vi "Dashboard Main.vi"() -> ()   [LabVIEW 2012]
uses:
  <vilib>/event_ctls.llb/eventvkey.ctl
  <vilib>/Utility/config.llb/Read Key (String).vi
  <vilib>/Utility/config.llb/Read Key (I32).vi
  <vilib>/Utility/config.llb/Write Key (String).vi
  <vilib>/Utility/config.llb/Write Key (I32).vi
  <vilib>/Utility/config.llb/NI_LVConfig.lvlib
panel:
  out "Mode":T1(ring)=enum."Auto Disabled"
  in  "Viewer":enum32{"Camera Image", "Variables"}(tab)
  out "Mbps":dbl format="%#.1g"
  in  "Enable":bool
  in  "DB Camera Config":bool
  out "Mbps":bool
  out "fps":dbl format="%#.1g"
  out "Image Error Message":string="Timeout in Camera Communications"
  out "Camera Image":T2(plugin-control)
  out "Camera Image 2":T2(plugin-control)
  in  "Camera Settings":T3={"Frame Rate"=15, "Compression"=30, "Size"=1} {"Frame Rate" scale=1.0..30.0; "Size" items=["640x480", "320x240", "160x120"]}
  out "Camera IP 2":string
  out "Camera IP":string
  out "fps 2":dbl format="%#.1g"
  out "Mbps 2":dbl format="%#.1g"
  in  "Enable 2":bool
  in  "FR":i32=15
  out "Tree":string(tree)
  in  "Dashboard Tab":enum32{"Operation", "Test", "Checklist"}(tab)
  in  "AutonSelector":bool[](array[boolean])
  in  "AutonRefresh":bool
  out "AutonFiles":string[](array[string])
  in  "Slider":dbl(slide) scale=0.0..100.0 scale format="%#_3g"
  in  "On/Off":bool caption="Solenoid"
  in  "Test Name":u16(ring) items=["Select the test to run...", "Example Test", "-------------------------------", "List of tests is built in robot code.", "Replace with your own automated tests."]
  in  "Test Tree":string(tree)
  in  "Motor":cluster{"Value":dbl, "Enable":bool} {"Value" scale=-1.0..1.0 scale format="%#_3g"}
  out "Progress":T4 {"Test Progress" scale=0.0..100.0}
  in  "Rev/Fwd":cluster{"Forward":bool, "Reverse":bool}
  in  "Ring":u16(ring) items=["Auto", "Fixed indoor", "Fixed outdoor 1", "Fixed outdoor 2", "Fixed fluorescent 1", "Fixed fluorescent 2", "Hold current"]
  in  "Listbox":i32(listbox)
  out "Robot IP":string
  out "Battery Value":dbl(slide) scale=0.0..14.0 scale format="%#_2e"
  out "Battery":sgl(graph)
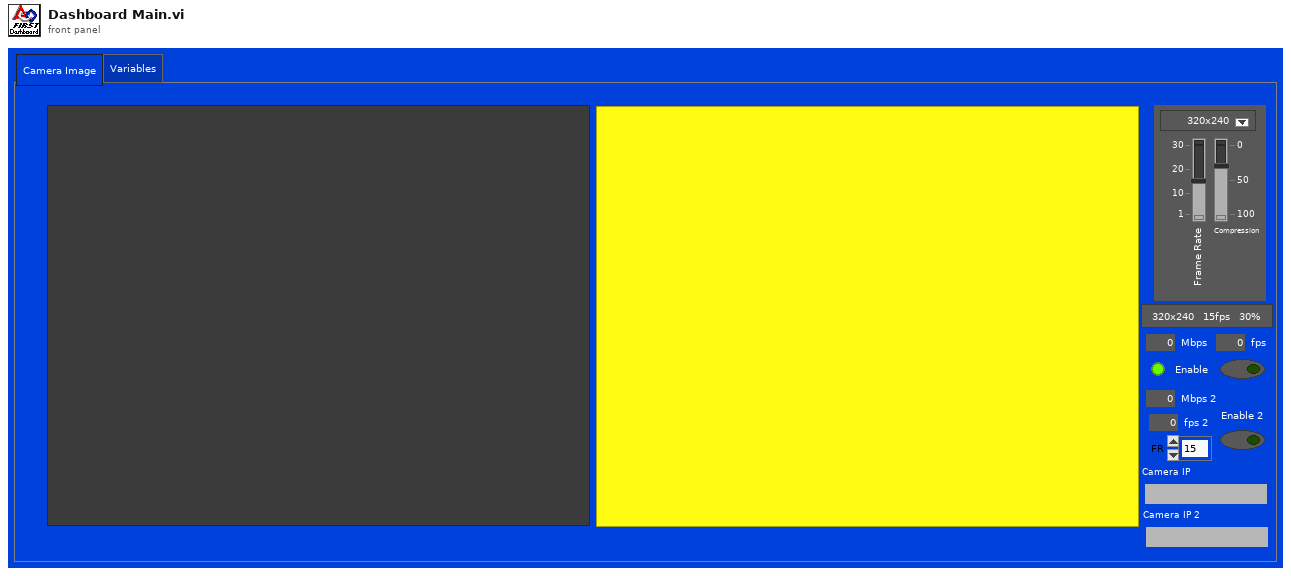
[diagram p1: front panel]
types:
  T1 = enum8{"Tele-Op Disabled", "Tele-Op Enabled", "Auto Disabled", "Auto Enabled", "Test Disabled", "Test Enabled", ""}
  T2 = typedef "IMAQ Image.ctl" = refnum<image>
  T3 = cluster{"Frame Rate":i32, "Compression":i32, "Size":u16}
  T4 = cluster{"Test Progress":u8, "Test Progress Text":string}
  T5 = typedef "Image Type" = u32
  T6 = cluster{"Competition mode":bool, "Robot Link":bool, "Autonomous":bool, "Enabled":bool, "E-Stop":bool, "Simulated":bool, "TestMode":bool, "Docked Window":bool}
  T7 = typedef "LVRectTypeDef.ctl" = cluster{"Left":i16, "Top":i16, "Right":i16, "Bottom":i16}
  T8 = typedef "NI_LVConfig.lvlib/Config Data RefNum.ctl" = refnum<k1>
  T9 = typedef "eventvkey.ctl" = enum16{"ASCII", "Enter", "Return", "Shift", "Ctrl", "Alt", "Cmd", "Opt", "Caps", "NumLock", "Clear", "Break", "Up", "Down", "Left", "Right", "Insert", "Delete", "Home", "End", "PageUp", "PageDown", "Escape", "Help", "Pause", "ScrollLock", "F1", "F2", "F3", "F4", "F5", "F6", "F7", "F8", "F9", "F10", "F11", "F12", "F13", "F14", "F15", "F16", "F17", "F18", "F19", "F20", "F21", "F22", "F23", "F24", "Play", "VolumeUp", "VolumeDown", "Mute", "Two Byte Char"}
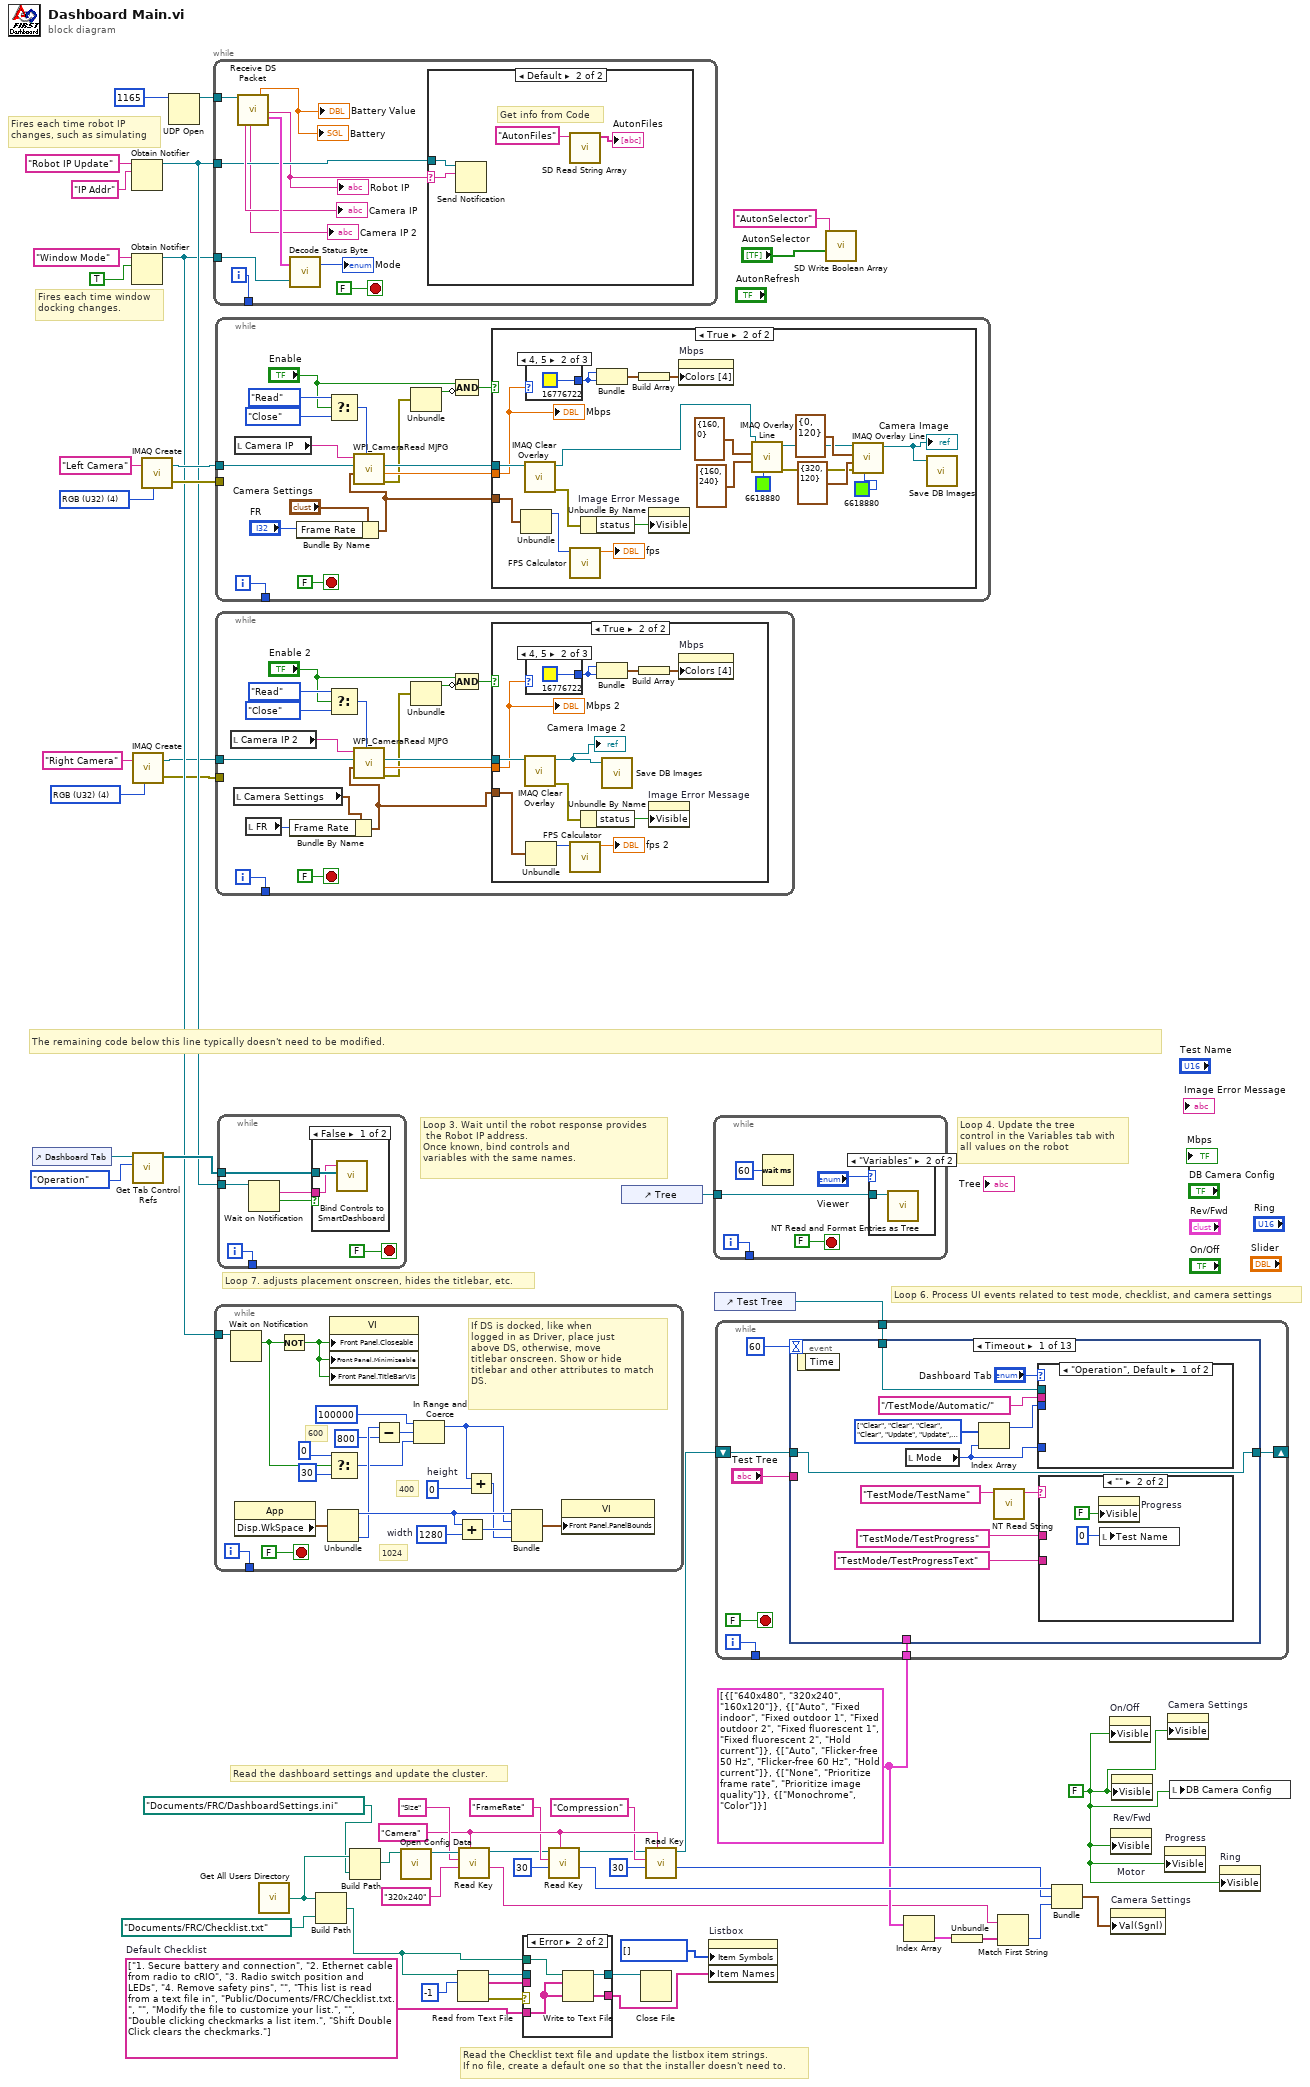
[diagram p0: block diagram]
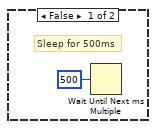
[diagram p2: hidden frame]
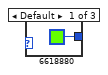
[diagram p3: hidden frame]
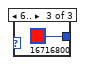
[diagram p4: hidden frame]
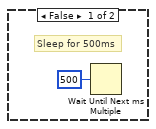
[diagram p6: hidden frame]
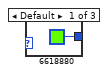
[diagram p7: hidden frame]
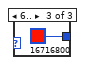
[diagram p8: hidden frame]
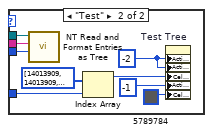
[diagram p10: hidden frame]
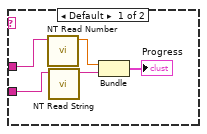
[diagram p11: hidden frame]
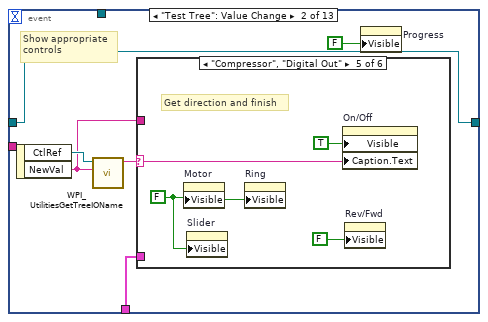
[diagram p12: hidden frame]
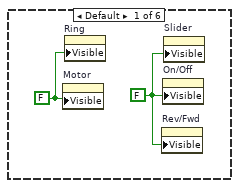
[diagram p13: hidden frame]
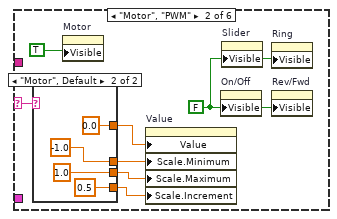
[diagram p14: hidden frame]
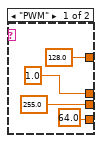
[diagram p15: hidden frame]
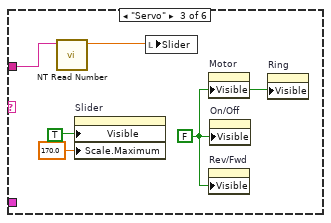
[diagram p16: hidden frame]
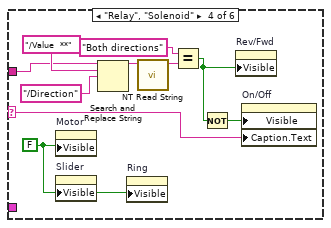
[diagram p17: hidden frame]
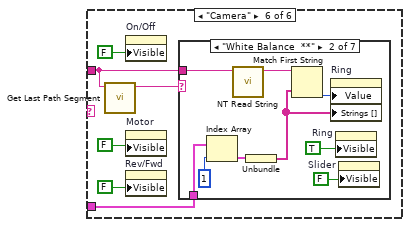
[diagram p18: hidden frame]
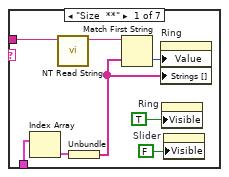
[diagram p19: hidden frame]
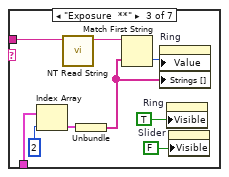
[diagram p20: hidden frame]
diagram:
  w5 = T5 4 items=["Grayscale (U8)", "Grayscale (I16)", "Grayscale (SGL)", "Complex (CSG)", "RGB (U32)", "HSL (U32)", "RGB (U64)"] ("Image Type")
  w27 = "Camera"
  w19 = cluster{string[]}[] [{["640x480", "320x240", "160x120"]}, {["Auto", "Fixed indoor", "Fixed outdoor 1", "Fixed outdoor 2", "Fixed fluorescent 1", "Fixed fluorescent 2", "Hold current"]}, {["Auto", "Flicker-free 50 Hz", "Flicker-free 60 Hz", "Hold current"]}, {["None", "Prioritize frame rate", "Prioritize image quality"]}, {["Monochrome", "Color"]}]
  w35 = string[] ["1. Secure battery and connection", "2. Ethernet cable from radio to cRIO", "3. Radio switch position and LEDs", "4. Remove safety pins", "", "This list is read from a text file in", "Public/Documents/FRC/Checklist.txt.", "", "Modify the file to customize your list.", "", "Double clicking checkmarks a list item.", "Shift Double Click clears the checkmarks."]  # Default Checklist
  w33 = FALSE ("Visible")
  w54 = T5 4 items=["Grayscale (U8)", "Grayscale (I16)", "Grayscale (SGL)", "Complex (CSG)", "RGB (U32)", "HSL (U32)", "RGB (U64)"] ("Image Type")
  # "Fires each time robot IP\nchanges, such as simulating"
  # "Fires each time window\ndocking changes."
  # "Read the Checklist text file and update the listbox item strings.\nIf no file, create a default one so that the installer doesn't need to."
  # "The remaining code below this line typically doesn't need to be modified."
  # "Loop 6. Process UI events related to test mode, checklist, and camera settings"
  # "Read the dashboard settings and update the cluster."
  # "Loop 4. Update the tree\ncontrol in the Variables tab with\nall values on the robot"
  # "Loop 3. Wait until the robot response provides\n the Robot IP address.\nOnce known, bind controls and\nvariables with the same names."
  # "Loop 7. adjusts placement onscreen, hides the titlebar, etc."
  n1 = control-ref of="Dashboard Tab"() -> (w49:refnum<vi>)
  n2 = Obtain Notifier(name (unnamed)="Robot IP Update", notification data type="IP Addr" ("name (unnamed)")) -> (notifier out=w46:refnum<notifier>)  [unwired: 2 in, 2 out]
  n3 = Obtain Notifier(name (unnamed)="Window Mode", notification data type=TRUE) -> (notifier out=w39:refnum<notifier>)  [unwired: 2 in, 2 out]
  n4 = call "IMAQ Create"("Image Name"="Right Camera", "Image Type"=w5) -> ("New Image"=w4:T2, "error out"=w3:errorcluster)  [unwired: 2 in, 1 out]
  n5 = call <vilib>:"Get Tab Control Refs.vi"("Page Index"=enum32{"Operation", "Test"}."Operation" ("Dashboard Tab"), "TabControl in"=w49) -> ("ControlsOnPage"=w50:refnum<vi>[])  [unwired: 9 in]
  n6 = call "IMAQ Create"("Image Name"="Left Camera", "Image Type"=w54) -> ("New Image"=w52:T2, "error out"=w51:errorcluster)  [unwired: 2 in, 1 out]
  n7 = UDP Open(11:u16 1165 ("port")) -> (port=w55:refnum<k16>)  [unwired: 2 in, 4 out]
  n8 = while {
    tunnel: w55 -> [w65]
    tunnel: w46 -> [w59]
    tunnel: w39 -> [w63]
    tunnel: [w60] -> _
    i -> [w60]
    stop <- FALSE stop-if-true
    n9 = call "Receive DS Packet.vi"("Recv Socket"=w65) -> ("Camera IP Address"=→"Camera IP":string, "Camera IP Address 2"=→"Camera IP 2":string, "Battery"=→"Battery" →"Battery Value":sgl, "Robot IP Address"=w58:string, "Status"=w66:T6)  [unwired: 8 in, 6 out]
    "Robot IP" <- w58
    n10 = call "Decode Status Byte.vi"("Window Mode Notifier"=w63, "Status"=w66) -> ("Mode"=→"Mode":T1)  [unwired: 1 out]
    n11 = case shown="Default" w58 {
      selector: w58 -> [_ w70]
      tunnel: w59 -> [_ w71]
      frame "0.0.0.0" {
        # "Robot not responding, don't poll the variables"
      }
      frame Default {
        # "Get info from Code"
        n12 = Send Notification(notification=w70, notifier=w71) -> ()  [unwired: 1 in, 2 out]
        n13 = call <vilib>:"SD Read String Array.vi"("Name"="AutonFiles") -> ("String Array"=→"AutonFiles":string[])  [unwired: 9 in, 1 out]
      }
    }
  }
  n14 = while {
    tunnel: w39 -> [w90]
    tunnel: [w88] -> _
    i -> [w88]
    stop <- FALSE stop-if-true
    w80 = 1280  # width
    w83 = 0  # height
    # "600"
    # "1024"
    # "400"
    # "If DS is docked, like when\nlogged in as Driver, place just\nabove DS, otherwise, move\ntitlebar onscreen. Show or hide\ntitlebar and other attributes to match\nDS."
    n15 = Wait on Notification(notifier=w90) -> (notification=w75:bool)  [unwired: 3 in, 3 out]
    n16 = property class="App"() -> ("Disp.WkSpace"=w86:T7)  [unwired: 2 in, 2 out]
    n17 = Not(x=w75) -> (.not. x?=w89:bool)
    n18 = Unbundle(w86) -> ("Left"=w84:i16, "Bottom"=w81:i16)  [unwired: 2 out]
    n19 = Select(t=0, s=w75, f=30) -> (s? t:f=w74:i32)
    n20 = property class="VI"("Front Panel.Closeable"=w89, "Front Panel.Minimizeable"=w89, "Front Panel.TitleBarVis"=w89) -> ()  [unwired: 2 in, 2 out]
    n21 = Subtract(x=w81, y=800) -> (x-y=w78:i32)
    n22 = In Range and Coerce(upper limit=100000, x=w78, lower limit=w74) -> (coerced(x)=w72:i32)  [unwired: 1 out]
    n23 = Add(x=w84, y=w80) -> (x+y=w85:i32)
    n24 = Add(x=w72, y=w83) -> (x+y=w82:i32)
    n25 = Bundle("Left"=w84, w72, w85, w82) -> (w87:cluster{"Left":i16, i32, i32, i32})  [unwired: 1 out]
    n26 = property class="VI"("Front Panel.PanelBounds"=w87) -> ()  [unwired: 2 in, 2 out]
  }
  n27 = while {
    tunnel: w52 -> [w104]
    tunnel: w51 -> [_]
    tunnel: [w106] -> _
    i -> [w106]
    stop <- FALSE stop-if-true
    n28 = local read "Camera IP"() -> (w105:string)
    n29 = Bundle By Name(cluster="Camera Settings", "Frame Rate"="FR") -> (w92:T3)
    n30 = Select(t=enum16{"Read", "Reopen", "Close"}."Read" ("Operation"), s="Enable", f=enum16{"Read", "Reopen", "Close"}."Close" ("Operation")) -> (s? t:f=w99:enum16{"Read", "Reopen", "Close"})
    n31 = call <vilib>:"WPI_CameraRead MJPG.vi"("Operation"=w99, "Camera Settings"=w92, "Image"=w104, "address"=w105) -> ("error out"=w98:errorcluster, "Bandwidth (kbps)"=w102:dbl, "Image Out"=w103:T2)  [unwired: 5 in]
    n32 = Unbundle(w98) -> ("status"=w96:bool)  [unwired: 2 out]
    n33 = Compound Arithmetic op=AND("Enable", invert w96) -> (w95:bool)
    n34 = case shown="True" w95 {
      tunnel: w92 -> [_ w120]
      tunnel: w103 -> [_ w123]
      tunnel: w102 -> [_ w122]
      frame False {
        # "Sleep for 500ms"
        n35 = Wait Until Next ms Multiple(millisecond multiple=u32 500) -> ()  [unwired: 1 out]
      }
      frame True {
        n36 = Unbundle(w120) -> ("Frame Rate"=w110:i32)  [unwired: 2 out]
        n37 = call "IMAQ Clear Overlay"("Image"=w123) -> ("error out"=w127:errorcluster, "Image Out"=w112:T2)  [unwired: 2 in, 7 out]
        n38 = case shown="4, 5" w122 {
          tunnel: [u32 6618880 ("Color Box") u32 16776722 ("Color Box") u32 16716800 ("Color Box")] -> w124
          frame Default {
          }
          frame 4, 5 {
          }
          frame 6.. {
          }
        }
        n39 = call "FPS Calculator.vi"("Average Count"=w110) -> ("fps"=→"fps":dbl)  [unwired: 10 in]
        n40 = Unbundle By Name(w127) -> ("status"=w128:bool)
        n41 = Bundle("Color Box"=w124, "Color Box"=w124) -> (w126:cluster{"Color Box":u32, "Color Box":u32})  [unwired: 1 out]
        n42 = Build Array(w126) -> (w125:cluster{"Color Box":u32, "Color Box":u32}[])
        n43 = property on="Image Error Message" class="Str"("Visible"=w128) -> ()  [unwired: 2 in, 2 out]
        n44 = property on="Mbps" class="Bool (strict)"("Colors [4]"=w125) -> ()  [unwired: 2 in, 2 out]
        n45 = call "IMAQ Overlay Line"("Color"=u32 6618880, "End Point"=cluster{"X":i32, "Y":i32} {"X"=160, "Y"=240}, "Start Point"=cluster{"X":i32, "Y":i32} {"X"=160, "Y"=0}, "Image"=w112) -> ("error out"=w117:errorcluster, "Image Out"=w116:T2)  [unwired: 6 in]
        n46 = call "IMAQ Overlay Line"("Color"=u32 6618880, "error in (no error)"=w117, "End Point"=cluster{"X":i32, "Y":i32} {"X"=320, "Y"=120}, "Start Point"=cluster{"X":i32, "Y":i32} {"X"=0, "Y"=120}, "Image"=w116) -> ("Image Out"=w111:T2)  [unwired: 5 in, 1 out]
        "Camera Image" <- w111
        n47 = call "Save DB Images.vi"("Image"=w111) -> ()  [unwired: 2 in, 1 out]
        "Mbps" <- w122
      }
    }
  }
  n48 = while {
    tunnel: w4 -> [w144]
    tunnel: [w146] -> _
    tunnel: w3 -> [_]
    i -> [w146]
    stop <- FALSE stop-if-true
    n49 = local read "Camera IP 2"() -> (w145:string)
    n50 = local read "Camera Settings"() -> (w133:T3)
    n51 = local read "FR"() -> (w134:i32)
    n52 = Bundle By Name(cluster=w133, "Frame Rate"=w134) -> (w132:T3)
    n53 = Select(t=enum16{"Read", "Reopen", "Close"}."Read" ("Operation"), s="Enable 2", f=enum16{"Read", "Reopen", "Close"}."Close" ("Operation")) -> (s? t:f=w139:enum16{"Read", "Reopen", "Close"})
    n54 = call <vilib>:"WPI_CameraRead MJPG.vi"("Operation"=w139, "Camera Settings"=w132, "Image"=w144, "address"=w145) -> ("error out"=w138:errorcluster, "Bandwidth (kbps)"=w142:dbl, "Image Out"=w143:T2)  [unwired: 5 in]
    n55 = Unbundle(w138) -> ("status"=w136:bool)  [unwired: 2 out]
    n56 = Compound Arithmetic op=AND("Enable 2", invert w136) -> (w135:bool)
    n57 = case shown="True" w135 {
      tunnel: w132 -> [_ w151]
      tunnel: w143 -> [_ w154]
      tunnel: w142 -> [_ w153]
      frame False {
        # "Sleep for 500ms"
        n58 = Wait Until Next ms Multiple(millisecond multiple=u32 500) -> ()  [unwired: 1 out]
      }
      frame True {
        n59 = call "IMAQ Clear Overlay"("Image"=w154) -> ("error out"=w158:errorcluster, "Image Out"=w149:T2)  [unwired: 2 in, 7 out]
        "Camera Image 2" <- w149
        n60 = case shown="4, 5" w153 {
          tunnel: [u32 6618880 ("Color Box") u32 16776722 ("Color Box") u32 16716800 ("Color Box")] -> w155
          frame Default {
          }
          frame 4, 5 {
          }
          frame 6.. {
          }
        }
        n61 = Unbundle(w151) -> ("Frame Rate"=w150:i32)  [unwired: 2 out]
        n62 = call "FPS Calculator.vi"("Average Count"=w150) -> ("fps"=→"fps 2":dbl)  [unwired: 10 in]
        n63 = Unbundle By Name(w158) -> ("status"=w159:bool)
        n64 = Bundle("Color Box"=w155, "Color Box"=w155) -> (w157:cluster{"Color Box":u32, "Color Box":u32})  [unwired: 1 out]
        n65 = call "Save DB Images.vi"("Image"=w149) -> ()  [unwired: 2 in, 1 out]
        n66 = Build Array(w157) -> (w156:cluster{"Color Box":u32, "Color Box":u32}[])
        n67 = property on="Image Error Message" class="Str"("Visible"=w159) -> ()  [unwired: 2 in, 2 out]
        n68 = property on="Mbps" class="Bool (strict)"("Colors [4]"=w156) -> ()  [unwired: 2 in, 2 out]
        "Mbps 2" <- w153
      }
    }
  }
  n69 = while {
    tunnel: w50 -> [w168]
    tunnel: w46 -> [w165]
    tunnel: [w163] -> _
    i -> [w163]
    stop <- FALSE stop-if-true
    n70 = Wait on Notification(notifier=w165) -> (notification=w164:string, timed out?=w166:bool)  [unwired: 3 in, 2 out]
    n71 = case shown="False" w166 {
      tunnel: w168 -> [w170 _]
      tunnel: w164 -> [w169 _]
      frame False {
        n72 = call <vilib>:"Bind Controls to SmartDashboard.vi"("Bound Control Refs"=w170, "Server IP Address"=w169) -> ()  [unwired: 10 in]
      }
      frame True {
      }
    }
  }
  n73 = call "Get All Users Directory.vi"() -> ("All User Path"=w32:path)
  n74 = Build Path(base path=w32, name or relative path=path "Documents/FRC/Checklist.txt") -> (appended path=w36:path)
  n75 = Build Path(base path=w32, name or relative path=path "Documents/FRC/DashboardSettings.ini") -> (appended path=w31:path)
  n76 = call <vilib>:"Open Config Data.vi"("configuration file path"=w31) -> ("refnum"=w30:T8)  [unwired: 8 in, 2 out]
  n77 = Read from Text File(file (use dialog)=w36, count=-1 ("timeout ms (25000)")) -> (refnum out=w14:refnum<file>, text=w37:string[], error out=w38:errorcluster)  [unwired: 2 in, 1 out]
  n78 = call-poly <vilib>:"Read Key.vi"("section"=w27, "default value"="320x240", "key"="Size", "refnum"=w30) -> ("value"=w17:string, "refnum out"=w12:T8)  [unwired: 2 in, 4 out]
  n79 = case shown="Error" w38 {
    tunnel: w37 -> [w172 _]
    tunnel: [w172 w174] -> w34
    tunnel: w35 -> [_ w174]
    tunnel: w36 -> [_ w175]
    tunnel: [w171 w173] -> w13
    tunnel: w14 -> [w171 _]
    frame No Error {
    }
    frame Error {
      n80 = Write to Text File(file (use dialog)=w175, text=w174) -> (refnum out=w173:refnum<file>)  [unwired: 2 in, 2 out]
    }
  }
  n81 = call-poly <vilib>:"Read Key.vi"("section"=w27, "default value"=30, "key"="FrameRate", "refnum"=w12) -> ("value"=w22:i32, "refnum out"=w11:T8)  [unwired: 1 in, 5 out]
  n82 = control-ref of="Tree"() -> (w8:refnum<vi>)
  n83 = Close File(refnum=w13) -> ()  [unwired: 1 in, 2 out]
  n84 = call-poly <vilib>:"Read Key.vi"("section"=w27, "default value"=30, "key"="Compression", "refnum"=w11) -> ("value"=w21:i32, "refnum out"=w9:T8)  [unwired: 1 in, 5 out]
  n85 = property on="Listbox" class="LstBox (strict)"("Item Symbols"=i32[] [], "Item Names"=w34) -> ()  [unwired: 2 in, 2 out]
  n86 = while {
    tunnel: [w177] -> _
    tunnel: w8 -> [w176]
    i -> [w177]
    stop <- FALSE stop-if-true
    n87 = Wait (ms)(milliseconds to wait=u32 60) -> ()  [unwired: 1 out]
    n88 = case shown="\"Variables\"" "Viewer" {
      tunnel: w176 -> [_ w181]
      frame Default {
      }
      frame "Variables" {
        n89 = call <vilib>:"NT Read and Format Entries as Tree.vi"("Tree Refnum"=w181) -> ()  [unwired: 9 in, 2 out]
      }
    }
  }
  n90 = control-ref of="Test Tree"() -> (w7:refnum<vi>)
  n91 = while {
    tunnel: w19 -> [w186]
    shift-right: [w185] -> _
    shift-left: w9 -> [w184]
    tunnel: [w183] -> _
    tunnel: w7 -> [w182]
    i -> [w183]
    stop <- FALSE stop-if-true
    n92 = event shown="[0] Timeout" {
      selector: _ -> [_ _ _ _ _ _ _ _ _ _ _ _ _]
      dyn-events: _ -> [_ _ _ _ _ _ _ _ _ _ _ _ _]
      timeout: u32 60 ("milliseconds to wait") -> [_ _ _ _ _ _ _ _ _ _ _ _ _]
      tunnel: w182 -> [w196 _ _ _ _ _ _ _ _ _ _ _ _]
      tunnel: "Test Tree" -> [_ _ _ _ _ _ _ _ w390 w398 w400 w404 w412]
      tunnel: w186 -> [_ w218 _ _ _ _ w354 w384 _ _ _ _ _]
      tunnel: [w190 w217 _ w320 w328 w340 w353 w377 w389 w396 w399 w403 w411] -> w185
      tunnel: w184 -> [w190 w217 _ w320 w328 w340 w352 w377 w389 w396 w399 w403 w411]
      event Timeout {
        w195 = enum16{"Update", "Clear"}[] [enum."Clear", enum."Clear", enum."Clear", enum."Clear", enum."Update", enum."Update", enum."Clear"] items=["Update", "Clear"]
        n93 = event-data() -> ()  [unwired: 1 in, 1 out]
        n94 = local read "Mode"() -> (w193:T1)
        n95 = Index Array(array=w195, index=w193) -> (element=w194:enum16{"Update", "Clear"})
        n96 = call <vilib>:"NT Read String.vi"("Name"="TestMode/TestName") -> ("String"=w199:string)  [unwired: 9 in, 1 out]
        n97 = case shown="\"Operation\", Default" "Dashboard Tab" {
          tunnel: w196 -> [_ w209]
          tunnel: "/TestMode/Automatic/" ("Name Pattern") -> [_ w208]
          tunnel: w194 -> [_ w207]
          tunnel: w193 -> [_ w205]
          frame "Operation", Default {
          }
          frame "Test" {
            w204 = -2 ("Active Item:Row Number")
            n98 = call <vilib>:"NT Read and Format Entries as Tree.vi"("Operation"=w207, "Name Pattern"=w208, "Tree Refnum"=w209) -> ()  [unwired: 7 in, 2 out]
            n99 = Index Array(array=u32[] [14013909, 14013909, 14013909, 14013909, 14013909, 16777215, 14013909], index=w205) -> (element=w203:u32)
            n100 = property on="Test Tree" class="Tree (strict)"("Active Item Row Number"=w204, "ActiveColNum"=w204, "CellBG"=w203, "Active Item Row Number"=-1 ("Active Item:Row Number"), "CellBG"=u32 5789784 ("Color Box")) -> ()  [unwired: 2 in, 2 out]
          }
        }
        n101 = case shown="\"\"" w199 {
          tunnel: "TestMode/TestProgress" ("Name") -> [w211 _]
          tunnel: "TestMode/TestProgressText" ("Name") -> [w210 _]
          frame Default {
            n102 = call <vilib>:"NT Read Number.vi"("Name"=w211) -> ("Numeric"=w212:dbl)  [unwired: 9 in, 1 out]
            n103 = call <vilib>:"NT Read String.vi"("Name"=w210) -> ("String"=w213:string)  [unwired: 9 in, 1 out]
            n104 = Bundle("Numeric"=w212, "String"=w213) -> (→"Progress":cluster{"Numeric":dbl, "String":string})  [unwired: 1 in]
          }
          frame "" {
            n105 = property on="Progress" class="Clust (strict)"("Visible"=FALSE) -> ()  [unwired: 2 in, 2 out]
            n106 = local write "Test Name"(u16 0) -> ()
          }
        }
      }
      event "Test Tree": Value Change {
        # "Show appropriate\ncontrols"
        n107 = event-data() -> ("CtlRef"=w221:refnum<vi>, "NewVal"=w219:string)  [unwired: 1 in]
        n108 = call <vilib>:"WPI_UtilitiesGetTreeIOName.vi"("NewVal"=w219, "TreeControl in"=w221) -> ("I/O Name"=w222:string)  [unwired: 9 in]
        n109 = case shown="\"Compressor\", \"Digital Out\"" w222 {
          selector: w222 -> [_ w229 _ w247 w256 _]
          tunnel: w219 -> [_ _ w244 w246 _ w263]
          tunnel: w218 -> [_ _ _ _ _ w262]
          frame Default {
            w224 = FALSE ("Visible")
            w223 = FALSE ("Visible")
            n110 = property on="Motor" class="Clust (strict)"("Visible"=w223) -> ()  [unwired: 2 in, 2 out]
            n111 = property on="Ring" class="Ring (strict)"("Visible"=w223) -> ()  [unwired: 2 in, 2 out]
            n112 = property on="Rev/Fwd" class="Clust (strict)"("Visible"=w224) -> ()  [unwired: 2 in, 2 out]
            n113 = property on="On/Off" class="Bool (strict)"("Visible"=w224) -> ()  [unwired: 2 in, 2 out]
            n114 = property on="Slider" class="Slide (strict)"("Visible"=w224) -> ()  [unwired: 2 in, 2 out]
          }
          frame "Motor", "PWM" {
            w230 = FALSE ("Visible")
            n115 = case shown="\"Motor\", Default" w229 {
              tunnel: [1.0 ("Value") -1.0 ("Value")] -> w228
              tunnel: [255.0 ("Value") 1.0 ("Value")] -> w227
              tunnel: [128.0 ("Value") 0.0 ("Value")] -> w226
              tunnel: [64.0 ("Value") 0.5 ("Value")] -> w225
              frame "PWM" {
              }
              frame "Motor", Default {
              }
            }
            n116 = property on="Motor" class="Clust (strict)"("Visible"=TRUE) -> ()  [unwired: 2 in, 2 out]
            n117 = property on="Value" class="Slide (strict)"("Value"=w226, "Scale.Minimum"=w228, "Scale.Maximum"=w227, "Scale.Increment"=w225) -> ()  [unwired: 2 in, 2 out]
            n118 = property on="On/Off" class="Bool (strict)"("Visible"=w230) -> ()  [unwired: 2 in, 2 out]
            n119 = property on="Slider" class="Slide (strict)"("Visible"=w230) -> ()  [unwired: 2 in, 2 out]
            n120 = property on="Ring" class="Ring (strict)"("Visible"=w230) -> ()  [unwired: 2 in, 2 out]
            n121 = property on="Rev/Fwd" class="Clust (strict)"("Visible"=w230) -> ()  [unwired: 2 in, 2 out]
          }
          frame "Servo" {
            w242 = FALSE ("Visible")
            n122 = call <vilib>:"NT Read Number.vi"("Name"=w244) -> ("Numeric"=w243:dbl)  [unwired: 9 in, 1 out]
            n123 = property on="Slider" class="Slide (strict)"("Visible"=TRUE, "Scale.Maximum"=170.0 ("Scale.Range:Maximum")) -> ()  [unwired: 2 in, 2 out]
            n124 = local write "Slider"(w243) -> ()
            n125 = property on="Motor" class="Clust (strict)"("Visible"=w242) -> ()  [unwired: 2 in, 2 out]
            n126 = property on="Rev/Fwd" class="Clust (strict)"("Visible"=w242) -> ()  [unwired: 2 in, 2 out]
            n127 = property on="On/Off" class="Bool (strict)"("Visible"=w242) -> ()  [unwired: 2 in, 2 out]
            n128 = property on="Ring" class="Ring (strict)"("Visible"=w242) -> ()  [unwired: 2 in, 2 out]
          }
          frame "Relay", "Solenoid" {
            w245 = FALSE ("Visible")
            n129 = property on="Motor" class="Clust (strict)"("Visible"=w245) -> ()  [unwired: 2 in, 2 out]
            n130 = property on="Slider" class="Slide (strict)"("Visible"=w245) -> ()  [unwired: 2 in, 2 out]
            n131 = Search and Replace String(input string=w246, search string="/Value  **", replace string="/Direction") -> (result string=w252:string)  [unwired: 5 in, 3 out]
            n132 = property on="Ring" class="Ring (strict)"("Visible"=w245) -> ()  [unwired: 2 in, 2 out]
            n133 = call <vilib>:"NT Read String.vi"("Name"=w252) -> ("String"=w250:string)  [unwired: 9 in, 1 out]
            n134 = Equal?(x="Both directions", y=w250) -> (x = y?=w248:bool)
            n135 = Not(x=w248) -> (.not. x?=w249:bool)
            n136 = property on="Rev/Fwd" class="Clust (strict)"("Visible"=w248) -> ()  [unwired: 2 in, 2 out]
            n137 = property on="On/Off" class="Bool (strict)"("Visible"=w249, "Caption.Text"=w247) -> ()  [unwired: 2 in, 2 out]
          }
          frame "Compressor", "Digital Out" {
            w255 = FALSE ("Visible")
            # "Get direction and finish"
            n138 = property on="Motor" class="Clust (strict)"("Visible"=w255) -> ()  [unwired: 2 in, 2 out]
            n139 = property on="Slider" class="Slide (strict)"("Visible"=w255) -> ()  [unwired: 2 in, 2 out]
            n140 = property on="Ring" class="Ring (strict)"("Visible"=w255) -> ()  [unwired: 2 in, 2 out]
            n141 = property on="On/Off" class="Bool (strict)"("Visible"=TRUE, "Caption.Text"=w256) -> ()  [unwired: 2 in, 2 out]
            n142 = property on="Rev/Fwd" class="Clust (strict)"("Visible"=FALSE) -> ()  [unwired: 2 in, 2 out]
          }
          frame "Camera" {
            n143 = call <vilib>:"Get Last Path Segment.vi"("String in"=w263) -> ("String out"=w264:string)  [unwired: 10 in]
            n144 = property on="On/Off" class="Bool (strict)"("Visible"=FALSE) -> ()  [unwired: 2 in, 2 out]
            n145 = property on="Motor" class="Clust (strict)"("Visible"=FALSE) -> ()  [unwired: 2 in, 2 out]
            n146 = property on="Rev/Fwd" class="Clust (strict)"("Visible"=FALSE) -> ()  [unwired: 2 in, 2 out]
            n147 = case shown="\"White Balance  **\"" w264 {
              tunnel: w263 -> [w270 w279 w288 w297 w306 _ w312]
              tunnel: w262 -> [w268 w276 w285 w294 w303 _ _]
              frame "Size  **" {
                n148 = Index Array(array=w268) -> (element=w267:cluster{string[]})  [unwired: 1 in]
                n149 = call <vilib>:"NT Read String.vi"("Name"=w270) -> ("String"=w269:string)  [unwired: 9 in, 1 out]
                n150 = Unbundle(w267) -> (w265:string[])
                n151 = Match First String(2:w265, 3:w269) -> (0:w266:i32)  [unwired: 1 out]
                n152 = property on="Ring" class="Ring (strict)"("Value"=w266, "Strings []"=w265) -> ()  [unwired: 2 in, 2 out]
                n153 = property on="Ring" class="Ring (strict)"("Visible"=TRUE) -> ()  [unwired: 2 in, 2 out]
                n154 = property on="Slider" class="Slide (strict)"("Visible"=FALSE) -> ()  [unwired: 2 in, 2 out]
              }
              frame "White Balance  **" {
                n155 = Index Array(array=w276, index=1) -> (element=w277:cluster{string[]})
                n156 = call <vilib>:"NT Read String.vi"("Name"=w279) -> ("String"=w278:string)  [unwired: 9 in, 1 out]
                n157 = Unbundle(w277) -> (w274:string[])
                n158 = Match First String(2:w274, 3:w278) -> (0:w273:i32)  [unwired: 1 out]
                n159 = property on="Ring" class="Ring (strict)"("Value"=w273, "Strings []"=w274) -> ()  [unwired: 2 in, 2 out]
                n160 = property on="Ring" class="Ring (strict)"("Visible"=TRUE) -> ()  [unwired: 2 in, 2 out]
                n161 = property on="Slider" class="Slide (strict)"("Visible"=FALSE) -> ()  [unwired: 2 in, 2 out]
              }
              frame "Exposure  **" {
                n162 = Index Array(array=w285, index=2) -> (element=w286:cluster{string[]})
                n163 = call <vilib>:"NT Read String.vi"("Name"=w288) -> ("String"=w287:string)  [unwired: 9 in, 1 out]
                n164 = Unbundle(w286) -> (w282:string[])
                n165 = Match First String(2:w282, 3:w287) -> (0:w283:i32)  [unwired: 1 out]
                n166 = property on="Ring" class="Ring (strict)"("Value"=w283, "Strings []"=w282) -> ()  [unwired: 2 in, 2 out]
                n167 = property on="Ring" class="Ring (strict)"("Visible"=TRUE) -> ()  [unwired: 2 in, 2 out]
                n168 = property on="Slider" class="Slide (strict)"("Visible"=FALSE) -> ()  [unwired: 2 in, 2 out]
              }
              frame "Exposure Priority  **" {
                n169 = Index Array(array=w294, index=3) -> (element=w295:cluster{string[]})
                n170 = call <vilib>:"NT Read String.vi"("Name"=w297) -> ("String"=w296:string)  [unwired: 9 in, 1 out]
                n171 = Unbundle(w295) -> (w291:string[])
                n172 = Match First String(2:w291, 3:w296) -> (0:w292:i32)  [unwired: 1 out]
                n173 = property on="Ring" class="Ring (strict)"("Value"=w292, "Strings []"=w291) -> ()  [unwired: 2 in, 2 out]
                n174 = property on="Ring" class="Ring (strict)"("Visible"=TRUE) -> ()  [unwired: 2 in, 2 out]
                n175 = property on="Slider" class="Slide (strict)"("Visible"=FALSE) -> ()  [unwired: 2 in, 2 out]
              }
              frame "Color Enable  **" {
                n176 = Index Array(array=w303, index=4) -> (element=w304:cluster{string[]})
                n177 = call <vilib>:"NT Read String.vi"("Name"=w306) -> ("String"=w305:string)  [unwired: 9 in, 1 out]
                n178 = Unbundle(w304) -> (w300:string[])
                n179 = Match First String(2:w300, 3:w305) -> (0:w301:i32)  [unwired: 1 out]
                n180 = property on="Ring" class="Ring (strict)"("Value"=w301, "Strings []"=w300) -> ()  [unwired: 2 in, 2 out]
                n181 = property on="Ring" class="Ring (strict)"("Visible"=TRUE) -> ()  [unwired: 2 in, 2 out]
                n182 = property on="Slider" class="Slide (strict)"("Visible"=FALSE) -> ()  [unwired: 2 in, 2 out]
              }
              frame Default {
                n183 = property on="Ring" class="Ring (strict)"("Visible"=FALSE) -> ()  [unwired: 2 in, 2 out]
                n184 = property on="Slider" class="Slide (strict)"("Visible"=FALSE) -> ()  [unwired: 2 in, 2 out]
              }
              frame "Brightness  **", "Color Level  **", "Compression  **", "FPS  **", "Sharpness  **" {
                n185 = call <vilib>:"NT Read Number.vi"("Name"=w312) -> ("Numeric"=w311:dbl)  [unwired: 9 in, 1 out]
                n186 = local write "Slider"(w311) -> ()
                n187 = property on="Slider" class="Slide (strict)"("Visible"=TRUE, "Scale.Maximum"=100.0 ("Scale.Range:Maximum")) -> ()  [unwired: 2 in, 2 out]
                n188 = property on="Ring" class="Ring (strict)"("Visible"=FALSE) -> ()  [unwired: 2 in, 2 out]
              }
            }
          }
        }
        n189 = property on="Progress" class="Clust (strict)"("Visible"=FALSE) -> ()  [unwired: 2 in, 2 out]
      }
      event "Test Name": Mouse Enter {
        # "Populate the ring with the list of tests"
        n190 = event-data() -> ()  [unwired: 1 in, 1 out]
        n191 = call <vilib>:"NT Read String Array.vi"("Name"="TestMode/TestList") -> ("String Array"=w319:string[])  [unwired: 9 in, 1 out]
        n192 = Build Array (concatenate)("Select the test to run...", w319) -> (w318:string[])
        n193 = property on="Test Name" class="Ring (strict)"("Strings []"=w318) -> ()  [unwired: 2 in, 2 out]
      }
      event "Test Name": Value Change {
        w321 = FALSE ("Visible")
        # "Tell the robot the test name to run"
        n194 = event-data() -> ("NewVal"=w325:u16)  [unwired: 1 in]
        n195 = property on="Test Name" class="Ring (strict)"() -> ("Strings []"=w326:string[])  [unwired: 2 in, 2 out]
        n196 = local write "Progress"(T4 {"Test Progress"=0, "Test Progress Text"=""} ("Progress")) -> ()
        n197 = Index Array(array=w326, index=w325) -> (element=w324:string)
        n198 = call <vilib>:"NT Write String.vi"("String"=w324, "Name"="TestMode/TestName") -> ()  [unwired: 9 in, 1 out]
        n199 = property on="Progress" class="Clust (strict)"("Visible"=TRUE) -> ()  [unwired: 2 in, 2 out]
        n200 = property on="Motor" class="Clust (strict)"("Visible"=w321) -> ()  [unwired: 2 in, 2 out]
        n201 = property on="Slider" class="Slide (strict)"("Visible"=w321) -> ()  [unwired: 2 in, 2 out]
        n202 = property on="On/Off" class="Bool (strict)"("Visible"=w321) -> ()  [unwired: 2 in, 2 out]
        n203 = property on="Rev/Fwd" class="Clust (strict)"("Visible"=w321) -> ()  [unwired: 2 in, 2 out]
        n204 = property on="Ring" class="Ring (strict)"("Visible"=w321) -> ()  [unwired: 2 in, 2 out]
      }
      event "Listbox": Double Click {
        n205 = event-data() -> ("PlatMods.Shift"=w329:bool, "Row"=w331:i32)  [unwired: 1 in]
        n206 = case shown="False" w329 {
          tunnel: w331 -> [w335 _]
          tunnel: 1 -> [w334 _]
          frame False {
            n207 = property on="Listbox" class="LstBox (strict)"() -> ("Item Symbols"=w333:i32[])  [unwired: 2 in, 2 out]
            n208 = Replace Array Subset(array=w333, new element=w334, index=w335) -> (w332:i32[])
            n209 = property on="Listbox" class="LstBox (strict)"("Item Symbols"=w332) -> ()  [unwired: 2 in, 2 out]
          }
          frame True {
            w336 = 0 ("Top Row")
            n210 = property on="Listbox" class="LstBox (strict)"() -> ("Number of Rows"=w338:u32)  [unwired: 2 in, 2 out]
            n211 = Initialize Array(0, w338) -> (w337:i32[])
            n212 = property on="Listbox" class="LstBox (strict)"("Top Row"=w336, "Value"=w336, "Item Symbols"=w337) -> ()  [unwired: 2 in, 2 out]
          }
        }
      }
      event "Listbox": Key Down {
        n213 = event-data() -> ("VKey"=w342:T9)  [unwired: 1 in]
        n214 = case shown="\"Left\", \"Right\"" w342 {
          selector: w342 -> [w347 _]
          tunnel: eventvkey."Left" ("VKey") -> [w345 _]
          frame "Left", "Right" {
            n215 = Equal?(x=w345, y=w347) -> (x = y?=w346:bool)
            n216 = Select(t=0, s=w346, f=1) -> (s? t:f=w348:i32)
            n217 = property on="Listbox" class="LstBox (strict)"() -> ("Item Symbols"=w351:i32[])  [unwired: 2 in, 2 out]
            n218 = Replace Array Subset(array=w351, new element=w348, index="Listbox") -> (w350:i32[])
            n219 = property on="Listbox" class="LstBox (strict)"("Item Symbols"=w350) -> ()  [unwired: 2 in, 2 out]
          }
          frame Default {
          }
        }
      }
      event "DB Camera Config": Value Change {
        n220 = event-data() -> ("NewVal"=w355:bool)  [unwired: 1 in]
        n221 = case shown="False" w355 {
          tunnel: w354 -> [w364 _]
          tunnel: [w357 w375] -> w353
          tunnel: w352 -> [w356 w375]
          frame False {
            w371 = "Camera"
            w374 = FALSE ("Visible")
            n222 = local read "Camera Settings"() -> (w363:T3)
            n223 = Index Array(array=w364) -> (element=w367:cluster{string[]})  [unwired: 1 in]
            n224 = Unbundle(w363) -> ("Frame Rate"=w362:i32, "Compression"=w361:i32, "Size"=w365:u16)
            n225 = Unbundle(w367) -> (w366:string[])
            n226 = Index Array(array=w366, index=w365) -> (element=w360:string)
            n227 = call-poly <vilib>:"Write Key.vi"("section"=w371, "value"=w360, "key"="Size", "refnum"=w356) -> ("refnum out"=w373:T8)  [unwired: 2 in, 5 out]
            n228 = call-poly <vilib>:"Write Key.vi"("section"=w371, "value"=w362, "key"="FrameRate", "refnum"=w373) -> ("refnum out"=w372:T8)  [unwired: 1 in, 6 out]
            n229 = property on="Camera Settings" class="Clust (strict)"("Visible"=w374) -> ()  [unwired: 2 in, 2 out]
            n230 = local write "DB Camera Config"(w374) -> ()
            n231 = call-poly <vilib>:"Write Key.vi"("section"=w371, "value"=w361, "key"="Compression", "refnum"=w372) -> ("refnum out"=w358:T8)  [unwired: 1 in, 6 out]
            n232 = call <vilib>:"Close Config Data.vi"("refnum"=w358) -> ("file path"=w359:path)  [unwired: 2 in, 8 out]
            n233 = call <vilib>:"Open Config Data.vi"("configuration file path"=w359) -> ("refnum"=w357:T8)  [unwired: 8 in, 2 out]
          }
          frame True {
            n234 = property on="Camera Settings" class="Clust (strict)"("Visible"=TRUE) -> ()  [unwired: 2 in, 2 out]
          }
        }
      }
      event "Camera Settings": Value Change {
        n235 = event-data() -> ("NewVal"=w388:T3)  [unwired: 1 in]
        n236 = Index Array(array=w384) -> (element=w383:cluster{string[]})  [unwired: 1 in]
        n237 = Unbundle(w388) -> ("Frame Rate"=w379:i32, "Compression"=w378:i32, "Size"=w381:u16)
        n238 = Unbundle(w383) -> (w382:string[])
        n239 = Index Array(array=w382, index=w381) -> (element=w380:string)
        n240 = Format Into String(format string="%s   %dfps   %d%%", w380, w379, w378) -> (resulting string=w385:string)  [unwired: 2 in, 1 out]
        n241 = Build Array(w385) -> (w386:string[])
        n242 = property on="DB Camera Config" class="Bool (strict)"("Strings [4]"=w386) -> ()  [unwired: 2 in, 2 out]
      }
      event "Motor.Enable": Value Change {
        n243 = event-data() -> ("NewVal"=w394:bool)  [unwired: 1 in]
        n244 = Unbundle("Motor") -> ("Value"=w393:dbl)  [unwired: 1 out]
        n245 = Select(t=w393, s=w394, f=0.0) -> (s? t:f=w391:dbl)
        n246 = call <vilib>:"NT Write Number.vi"("Numeric"=w391, "Name"=w390) -> ()  [unwired: 9 in, 1 out]
      }
      event "Slider": Value Change {
        n247 = event-data() -> ("NewVal"=w397:dbl)  [unwired: 1 in]
        n248 = call <vilib>:"NT Write Number.vi"("Numeric"=w397, "Name"=w398) -> ()  [unwired: 9 in, 1 out]
      }
      event "On/Off": Value Change {
        n249 = event-data() -> ("NewVal"=w402:bool)  [unwired: 1 in]
        n250 = Boolean To (0,1)(Boolean=w402) -> (0, 1=w401:i16)
        n251 = call <vilib>:"NT Write Number.vi"("Numeric"=w401, "Name"=w400) -> ()  [unwired: 9 in, 1 out]
      }
      event "Rev/Fwd": Value Change {
        n252 = event-data() -> ("NewVal.Forward"=w410:bool, "NewVal.Reverse"=w409:bool)  [unwired: 1 in]
        n253 = Boolean To (0,1)(Boolean=w410) -> (0, 1=w406:i16)
        n254 = Boolean To (0,1)(Boolean=w409) -> (0, 1=w408:i16)
        n255 = Negate(x=w408) -> (-x=w407:i16)
        n256 = Add(x=w406, y=w407) -> (x+y=w405:i16)
        n257 = call <vilib>:"NT Write Number.vi"("Numeric"=w405, "Name"=w404) -> ()  [unwired: 9 in, 1 out]
      }
      event "Ring": Value Change {
        n258 = event-data() -> ("NewVal"=w414:u16)  [unwired: 1 in]
        n259 = property on="Ring" class="Ring (strict)"() -> ("Strings []"=w415:string[])  [unwired: 2 in, 2 out]
        n260 = Index Array(array=w415, index=w414) -> (element=w413:string)
        n261 = call <vilib>:"NT Write String.vi"("String"=w413, "Name"=w412) -> ()  [unwired: 9 in, 1 out]
      }
    }
  }
  n262 = call <vilib>:"SD Write Boolean Array.vi"("Boolean Array"="AutonSelector", "Name"="AutonSelector") -> ()  [unwired: 8 in, 2 out]
  n263 = Index Array(array=w19) -> (element=w20:cluster{string[]})  [unwired: 1 in]
  n264 = Unbundle(w20) -> (w18:string[])
  n265 = Match First String(2:w18, 3:w17) -> (0:w16:i32)  [unwired: 1 out]
  n266 = Bundle("value"=w22, "value"=w21, "index"=w16) -> (w10:cluster{"value":i32, "value":i32, "index":i32})  [unwired: 1 out]
  n267 = property on="On/Off" class="Bool (strict)"("Visible"=w33) -> ()  [unwired: 2 in, 2 out]
  n268 = property on="Motor" class="Clust (strict)"("Visible"=w33) -> ()  [unwired: 2 in, 2 out]
  n269 = property on="Camera Settings" class="Clust (strict)"("Val(Sgnl)"=w10) -> ()  [unwired: 2 in, 2 out]
  n270 = property on="Rev/Fwd" class="Clust (strict)"("Visible"=w33) -> ()  [unwired: 2 in, 2 out]
  n271 = property on="Progress" class="Clust (strict)"("Visible"=w33) -> ()  [unwired: 2 in, 2 out]
  n272 = property on="Camera Settings" class="Clust (strict)"("Visible"=w33) -> ()  [unwired: 2 in, 2 out]
  n273 = local write "DB Camera Config"(w33) -> ()
  n274 = property on="Ring" class="Ring (strict)"("Visible"=w33) -> ()  [unwired: 2 in, 2 out]
